vi "探头测量量程设置.vi"(7 "校准参数":u16(ring) caption="校准参数：" items=["pH", "DO", "浊度", "电导率", "叶绿素a", "藻密度", "ORP", "DO2"], 8 "error in (no error)":errorcluster caption="错误输入（无错误）", 11 "测量量程设置":u16) -> (0 "error out":errorcluster caption="错误输出")   [LabVIEW 2016, in "斯坦道多参数.lvlib"]
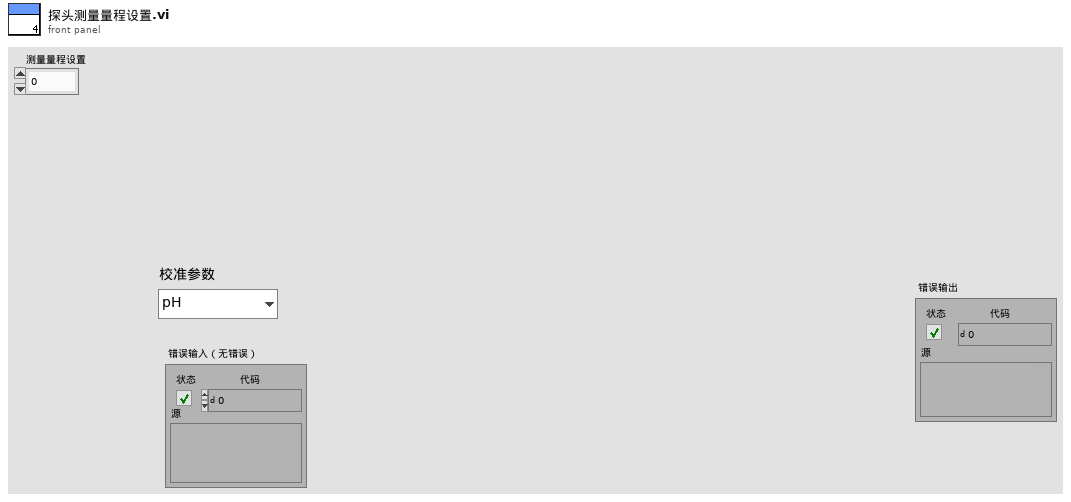
[diagram p1: front panel]
types:
  T1 = typedef "斯坦道多参数.lvlib/探头类型.ctl" = enum16{"禹山", "国弘", "纳清", "STD"}
  T2 = enum16{"null", "pH", "DO", "浊度", "电导率", "叶绿素a", "藻密度"}
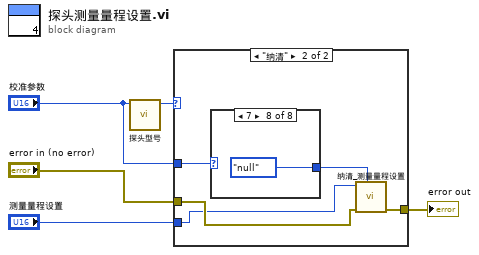
[diagram p0: block diagram]
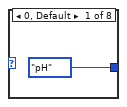
[diagram p3: hidden frame]
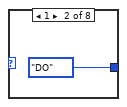
[diagram p4: hidden frame]
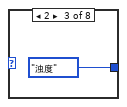
[diagram p5: hidden frame]
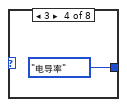
[diagram p6: hidden frame]
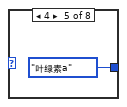
[diagram p7: hidden frame]
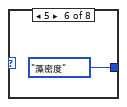
[diagram p8: hidden frame]
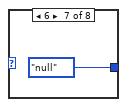
[diagram p9: hidden frame]
diagram:
  n1 = call "探头型号.vi"("校准参数"="校准参数") -> ("探头型号"=w5:T1)  [unwired: 8 in, 2 out]
  n2 = case shown="\"纳清\"" w5 {
    tunnel: "校准参数" -> [_ w11]
    tunnel: "error in (no error)" -> [w6 w8]
    tunnel: [w6 w9] -> w2
    tunnel: "测量量程设置" -> [_ w7]
    frame "禹山", Default {
    }
    frame "纳清" {
      n3 = case shown="7" w11 {
        tunnel: [T2."pH" ("探头") T2."DO" ("探头") T2."浊度" ("探头") T2."电导率" ("探头") T2."叶绿素a" ("探头") T2."藻密度" ("探头") T2."null" ("探头") T2."null" ("探头")] -> w10
        frame 0, Default {
        }
        frame 1 {
        }
        frame 2 {
        }
        frame 3 {
        }
        frame 4 {
        }
        frame 5 {
        }
        frame 6 {
        }
        frame 7 {
        }
      }
      n4 = call "纳清_测量量程设置.vi"("探头"=w10, "error in (no error)"=w8, "测量量程设置"=w7) -> ("error out"=w9:errorcluster)  [unwired: 8 in]
    }
  }
  "error out" <- w2
